vi "mqttBuildConnectFlagByte.vi"(0 "mqtt in":refnum<class "mqtt.lvclass">, 11 "error in (no error)":errorcluster) -> (4 "mqtt out":refnum<class "mqtt.lvclass">, 8 "connFlagByte out":u8, 15 "error out":errorcluster)   [LabVIEW 2021, in "mqtt.lvclass"]
uses:
  mqtt.lvclass
  mqtt.lvclass/mqtt.ctl
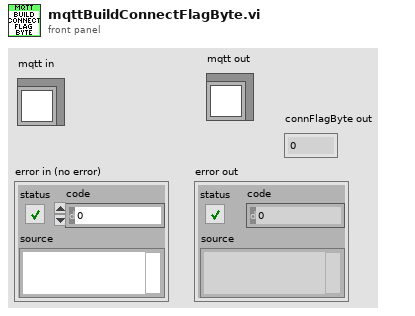
[diagram p1: front panel]
types:
  T1 = enum8{"At most once", "At least once", "Exactly once", "Reserved"}
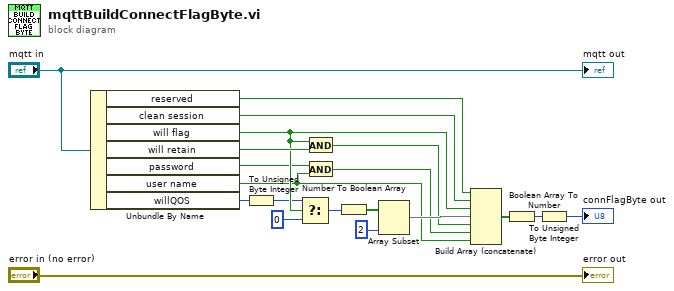
[diagram p0: block diagram]
diagram:
  n1 = Unbundle By Name("mqtt in") -> ("reserved"=w18:bool, "clean session"=w19:bool, "will flag"=w9:bool, "will retain"=w11:bool, "password"=w4:bool, "user name"=w3:bool, "willQOS"=w8:T1)
  n2 = To Unsigned Byte Integer(number=w8) -> (unsigned 8bit integer=w7:u8)
  n3 = Select(t=w7, s=w9, f=u8 0) -> (s? t:f=w6:u8)
  n4 = And(x=w9, y=w11) -> (x .and. y?=w10:bool)
  n5 = And(x=w4, y=w3) -> (x .and. y?=w2:bool)
  n6 = Number To Boolean Array(number=w6) -> (Boolean array=w17:bool[])
  n7 = Array Subset(array=w17, length=2) -> (w15:bool[])  [unwired: 1 in]
  n8 = Build Array (concatenate)(w18, w19, w9, w15, w10, w2, w3) -> (w14:bool[])
  n9 = Boolean Array To Number(Boolean array=w14) -> (number=w13:u32)
  n10 = To Unsigned Byte Integer(number=w13) -> (unsigned 8bit integer=→"connFlagByte out":u8)
  "error out" <- "error in (no error)"
  "mqtt out" <- "mqtt in"
